vi "Test Keys.vi"(8 "error in (no error)":errorcluster, 11 "VGC in":refnum<class "PL Inficon VGC.lvclass">) -> (0 "error out":errorcluster, 2 "keys":T1 {"key 4" items=["not pushed", "pushed"]; "key 3" items=["not pushed", "pushed"]; "key 2" items=["not pushed", "pushed"]; "key 1" items=["not pushed", "pushed"]}, 3 "VGC out":refnum<class "PL Inficon VGC.lvclass">)   [LabVIEW 2015, in "PL Inficon VGC.lvclass"]
doc: "Tests keys."
uses:
  PL Inficon VGC.lvclass
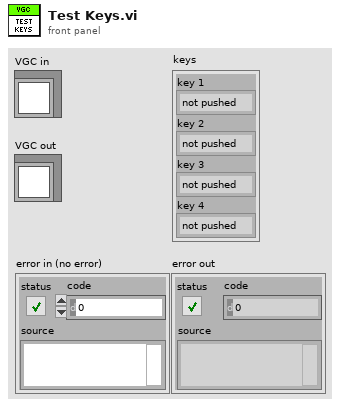
[diagram p1: front panel]
types:
  T1 = cluster{"key 1":u16, "key 2":u16, "key 3":u16, "key 4":u16}
  T2 = cluster{"[0]":i32, "[1]":i32, "[2]":i32, "[3]":i32}
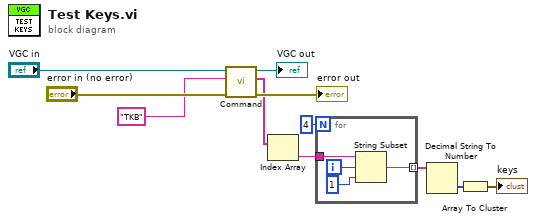
[diagram p0: block diagram]
diagram:
  n1 = call "Command.vi"("error in (no error)"="error in (no error)", "command"="TKB", "VGC in"="VGC in") -> ("error out"=→"error out":errorcluster, "response data"=w5:string[], "VGC out"=→"VGC out":refnum<class "PL Inficon VGC.lvclass">)  [unwired: 6 in]
  n2 = Index Array(array=w5) -> (element=w4:string)  [unwired: 1 in]
  n3 = for {
    N: 4 -> [_]
    tunnel: w4 -> [w14]
    tunnel: [w12] -> w3 mode=indexing
    i -> [w15]
    n4 = String Subset(string=w14, offset (0)=w15, length (rest)=1 ("length (rest)")) -> (substring=w12:string)
  }
  n5 = Decimal String To Number(string=w3) -> (number=w2:i32[])  [unwired: 2 in, 1 out]
  n6 = Array To Cluster(array=w2) -> (cluster=→"keys":T2)
